vi "CALC_Angle_from_center_towards_mouse_(arr).vi"(2 "Mouse Yc":dbl[](array[numeric]), 3 "Mouse Xc":dbl[](array[numeric])) -> (0 "abs(theta) < pi, rad":dbl[](array[numeric]), 1 "theta, rad":dbl[](array[numeric]))   [LabVIEW 2018, in "Tracker.lvlib"]
uses:
  Tracker.lvlib
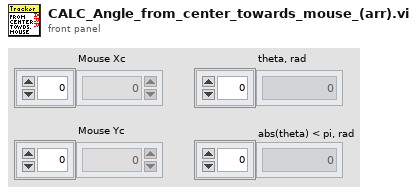
[diagram p1: front panel]
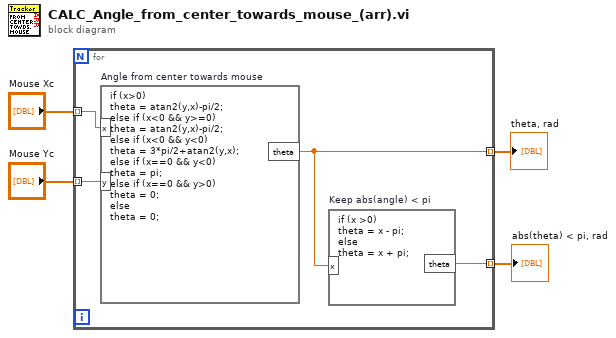
[diagram p0: block diagram]
diagram:
  n1 = for {
    tunnel: "Mouse Xc" -> [w8] mode=indexing
    tunnel: "Mouse Yc" -> [w7] mode=indexing
    tunnel: [w6] -> w2 mode=indexing
    tunnel: [w5] -> w1 mode=indexing
    n2 = formula code="if (x>0)\ntheta = atan2(y,x)-pi/2;\nelse if (x<0 && y>=0)\ntheta = atan2(y,x)-pi/2;\nelse if (x<0 && y<0)\ntheta = 3*pi/2+atan2(y,x);\nelse if (x==0 && y<0)\ntheta = pi;\nelse if (x==0 && y>0)\ntheta = 0;\nelse\ntheta = 0;" "Angle from center towards mouse"("x"=w8, "y"=w7) -> ("theta"=w6:dbl)
    n3 = formula code="if (x >0)\ntheta = x - pi;\nelse\ntheta = x + pi;" "Keep abs(angle) < pi"("x"=w6) -> ("theta"=w5:dbl)
  }
  "theta, rad" <- w2
  "abs(theta) < pi, rad" <- w1
